vi "Get_Target_Type.vi"(8 "error in (no error)":errorcluster, 9 "install path":string, 10 "default install path":string, 11 "userFolder in":refnum<class "userFolder.lvclass">) -> (0 "error out":errorcluster, 1 "path for target type":T1=68 items=["Relative to default installation directory"=68, "Root directory on first partition"=70, "Relative to directory table key"=82, "Absolute path to file"=65], 2 "path for target":string, 3 "userFolder out":refnum<class "userFolder.lvclass">)   [LabVIEW 2020, in "userFolder.lvclass"]
uses:
  <vilib>/AppBuilder/IB_Classes/Destination/userFolder/userFolder.lvclass
  <vilib>/AppBuilder/IB_Classes/Destination/userFolder/userFolder.lvclass/userFolder.ctl
  <vilib>/AppBuilder/IB_Classes/Destination/IB_Destination.lvclass
  AppLibs/distkit/MDF/NIMdf.llb/MDFBDPAddFilePathType.ctl
  AppLibs/distkit/MDF/NI_MDF.lvlib
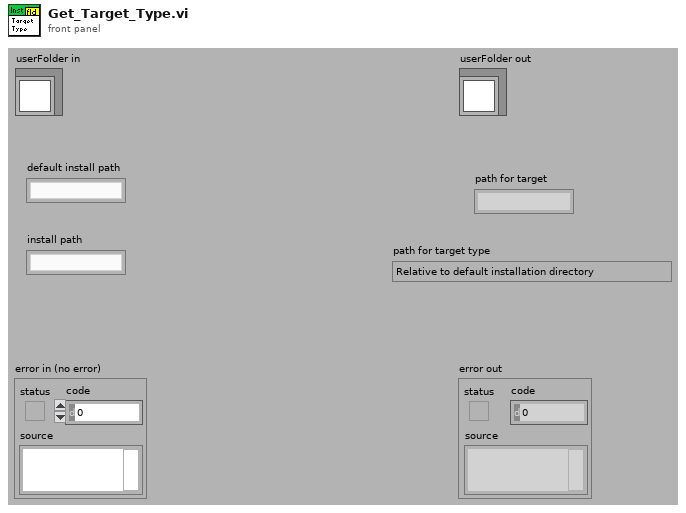
[diagram p1: front panel]
types:
  T1 = typedef "NI_MDF.lvlib/MDFBDPAddFilePathType.ctl" = i32
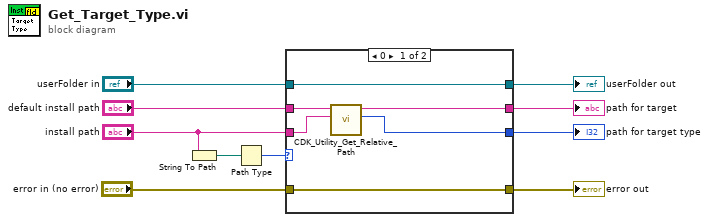
[diagram p0: block diagram]
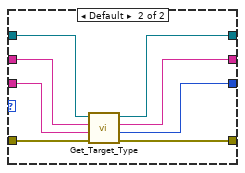
[diagram p2: hidden frame]
diagram:
  n1 = String To Path(string="install path") -> (path=w1:path)
  n2 = Path Type(1:w1) -> (0:w2:i16)
  n3 = case shown="0" w2 {
    tunnel: [w11 w17] -> w10
    tunnel: "error in (no error)" -> [w16 w24]
    tunnel: "install path" -> [w13 w19]
    tunnel: [w12 w18] -> w8
    tunnel: [w16 w23] -> w7
    tunnel: [w15 w21] -> w5
    tunnel: "userFolder in" -> [w15 w22]
    tunnel: "default install path" -> [w14 w20]
    frame 0 {
      n4 = call <resource>:"CDK_Utility_Get_Relative_Path.vi"("install path"=w13, "default install path"=w14) -> ("path for target type"=w11:T1, "path for target"=w12:string)  [unwired: 8 in]
    }
    frame Default {
      n5 = call-parent "Get_Target_Type.vi"("error in (no error)"=w24, "install path"=w19, "default install path"=w20, "IB_Destination in"=w22) -> ("error out"=w23:errorcluster, "path for target type"=w17:T1, "path for target"=w18:string, "IB_Destination out"=w21:refnum<class "userFolder.lvclass">)  [unwired: 4 in]
    }
  }
  "error out" <- w7
  "userFolder out" <- w5
  "path for target type" <- w10
  "path for target" <- w8
